vi "sigmoid.vi"(1 "Beta":dbl=1.0, 2 "input":dbl[](array[numeric])) -> (0 "output":dbl[](array[numeric]))   [LabVIEW 2009]
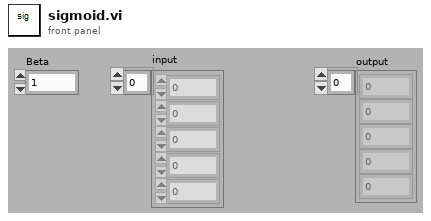
[diagram p1: front panel]
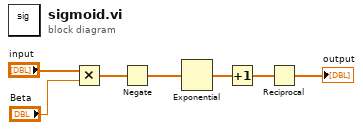
[diagram p0: block diagram]
diagram:
  n1 = Multiply(x="input", y="Beta") -> (x*y=w5:dbl[])
  n2 = Negate(x=w5) -> (-x=w4:dbl[])
  n3 = Exponential(1:w4) -> (0:w3:dbl[])
  n4 = Increment(x=w3) -> (x+1=w2:dbl[])
  n5 = Reciprocal(x=w2) -> (1/x=→"output":dbl[])
